vi "UpdateImage.vi"(8 "error in (no error)":errorcluster, 10 "JSON":string, 11 "WebSocket in":refnum<class "WebSocket.lvclass">) -> (0 "error out":errorcluster, 3 "WebSocket out":refnum<class "WebSocket.lvclass">)   [LabVIEW 2021, in "WebSocket.lvlib" / "WebSocket.lvclass"]
uses:
  WebSocket.lvclass
  Models/ImageResultModel.ctl
  55afc4ac-0a46-4e48-b16e-7859865e75a0.vi
  b0fb79d3-ebc5-46e5-b202-b11dbd438a97.vi
  <vilib>/JDP Science/JSONtext/JSON text to Variant.vi
  <vilib>/JDP Science/JSONtext/Variant to JSON Text.vi
  <vilib>/JDP Science/JSONtext/LVClass Serializer/JSONtext LVClass Serializer.lvclass
panel:
  out "x-y":u32
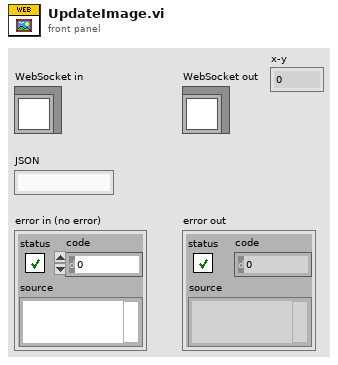
[diagram p1: front panel]
types:
  T1 = typedef "ImageResultModel.ctl" = cluster{"image":string, "pass":bool, "class":string, "time":dbl}
  T2 = cluster{"type":string, "imageResults":T1[], "ct":dbl, "uph":dbl}
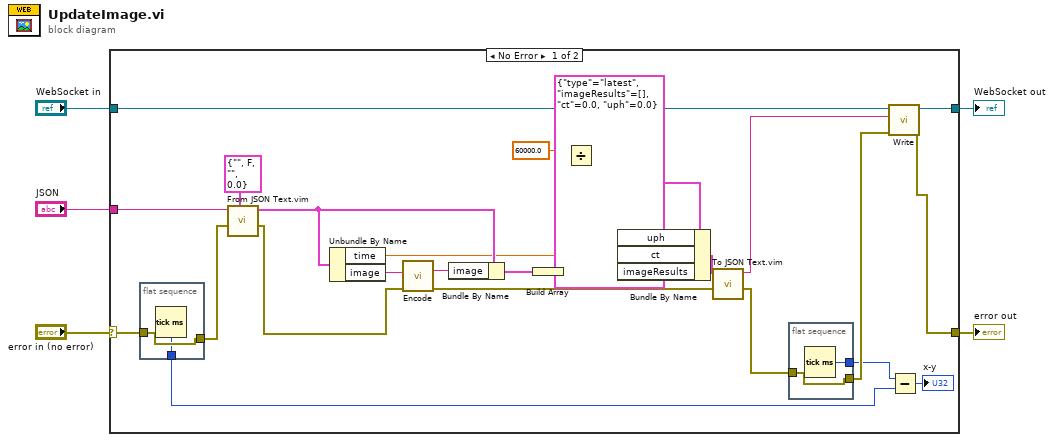
[diagram p0: block diagram]
diagram:
  n1 = case shown="No Error" "error in (no error)" {
    selector: "error in (no error)" -> [w24 w36]
    tunnel: [w28 w36] -> w4
    tunnel: [w27 w35] -> w2
    tunnel: "WebSocket in" -> [w29 w35]
    tunnel: "JSON" -> [w26 _]
    frame No Error {
      n2 = flat-sequence {
        tunnel: w24 -> [w34]
        tunnel: [w34] -> w23
        tunnel: [w33] -> w20
        frame #0 {
          n3 = Tick Count (ms)() -> (millisecond timer value=w33:u32)
        }
      }
      n4 = call "From JSON Text.vim"("Data Type and Default Value"=T1 {"image"="", "pass"=FALSE, "class"="", "time"=0.0} ("Cluster"), "error in (no error)"=w23, "JSON"=w26) -> ("error out"=w25:errorcluster, "Data out"=w17:T1)  [unwired: 7 in]
      n5 = Unbundle By Name(w17) -> ("time"=w8:dbl, "image"=w16:string)
      n6 = call "Encode.vi"("error in (no error)"=w25, "string in (not encoded)"=w16) -> ("error out"=w13:errorcluster, "string out (base64-encoded)"=w15:string)  [unwired: 8 in]
      n7 = Bundle By Name(cluster=w17, "image"=w15) -> (w10:T1)
      n8 = Build Array(w10) -> (w9:T1[])
      n9 = Divide(x=60000.0, y=w8) -> (x/y=w6:dbl)
      n10 = Bundle By Name(cluster=T2 {"type"="latest", "imageResults"=[], "ct"=0.0, "uph"=0.0}, "uph"=w6, "ct"=w8, "imageResults"=w9) -> (w14:T2)
      n11 = call "To JSON Text.vim"("error in (no error)"=w13, "Anything"=w14) -> ("error out"=w12:errorcluster, "<JSON>"=w11:string)  [unwired: 8 in]
      n12 = flat-sequence {
        tunnel: w12 -> [w32]
        tunnel: [w32] -> w22
        tunnel: [w31] -> w21
        frame #0 {
          n13 = Tick Count (ms)() -> (millisecond timer value=w31:u32)
        }
      }
      n14 = call "Write.vi"("error in (no error)"=w22, "Write"=w11, "WebSocket in"=w29) -> ("error out"=w28:errorcluster, "WebSocket out"=w27:refnum<class "WebSocket.lvclass">)  [unwired: 7 in]
      n15 = Subtract(x=w21, y=w20) -> (x-y=→"x-y":u32)
    }
    frame Error {
    }
  }
  "error out" <- w4
  "WebSocket out" <- w2
